vi "Read primaryAttackerId.vi"(8 "error in (no error)":errorcluster, 11 "SupportAttackerRole in":refnum<class "SupportAttackerRole.lvclass">) -> (0 "error out":errorcluster, 2 "primaryAttackerId":dbl, 3 "SupportAttackerRole out":refnum<class "SupportAttackerRole.lvclass">)   [LabVIEW 2023, in "SupportAttackerRole.lvclass"]
uses:
  SupportAttackerRole.lvclass
  SupportAttackerRole.lvclass/SupportAttackerRole.ctl
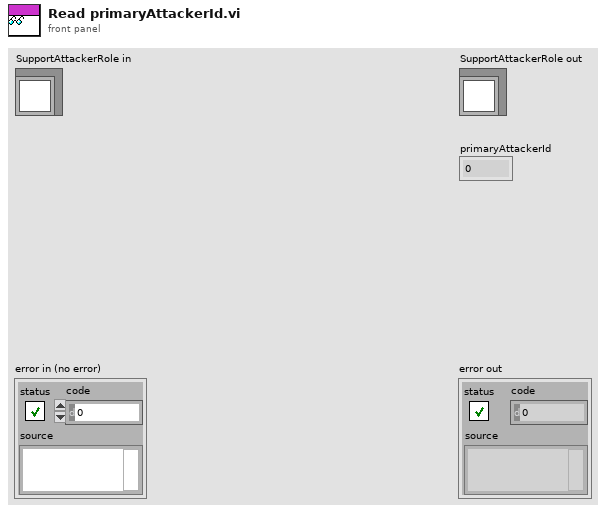
[diagram p1: front panel]
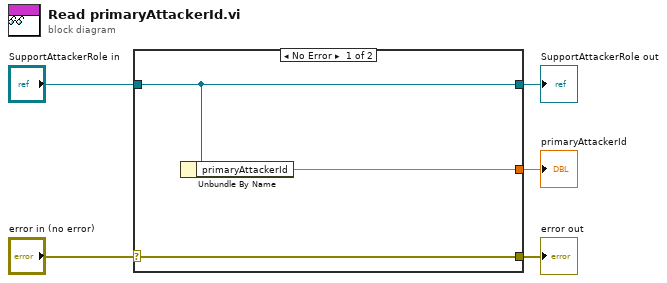
[diagram p0: block diagram]
diagram:
  n1 = case shown="No Error" "error in (no error)" {
    selector: "error in (no error)" -> [w8 w9]
    tunnel: [w8 w9] -> w4
    tunnel: [w7 w10] -> w2
    tunnel: "SupportAttackerRole in" -> [w7 w10]
    tunnel: [w6 _] -> w1
    frame No Error {
      n2 = Unbundle By Name(w7) -> ("primaryAttackerId"=w6:dbl)
    }
    frame Error {
    }
  }
  "error out" <- w4
  "SupportAttackerRole out" <- w2
  "primaryAttackerId" <- w1
